vi "DetectIon.vi"(10 "Samples per averaging\nblock":i32=100 min=1 step=1, 11 "Threshold":u32) -> (3 "Ion":bool)   [LabVIEW 2012]
uses:
  <vilib>/DAQmx/read.llb/DAQmx Read (Counter U32 1Chan 1Samp).vi
  <vilib>/DAQmx/create/channels.llb/DAQmx Create Channel (CI-Count Edges).vi
  <vilib>/DAQmx/configure/timing.llb/DAQmx Timing (Sample Clock).vi
  <vilib>/Analysis/baseanly.llb/Mean (DBL).vi
  <vilib>/DAQmx/miscellaneous.llb/DAQmx Fill In Error Info.vi
  <resource>/objmgr/daqmx.rc
  <vilib>/Analysis/NI_AALBase.lvlib
panel:
  out "Mean":dbl format="%0.2f"
  out "Variance":dbl format="%0.2f"
  out "Mean/Variance":dbl
  out "Counts":u32
  in  "Sample rate":dbl=50.0 format="%0.2f"
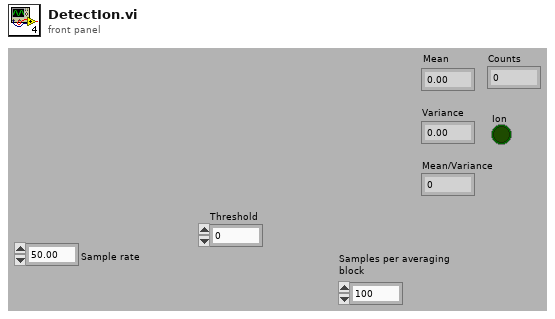
[diagram p1: front panel]
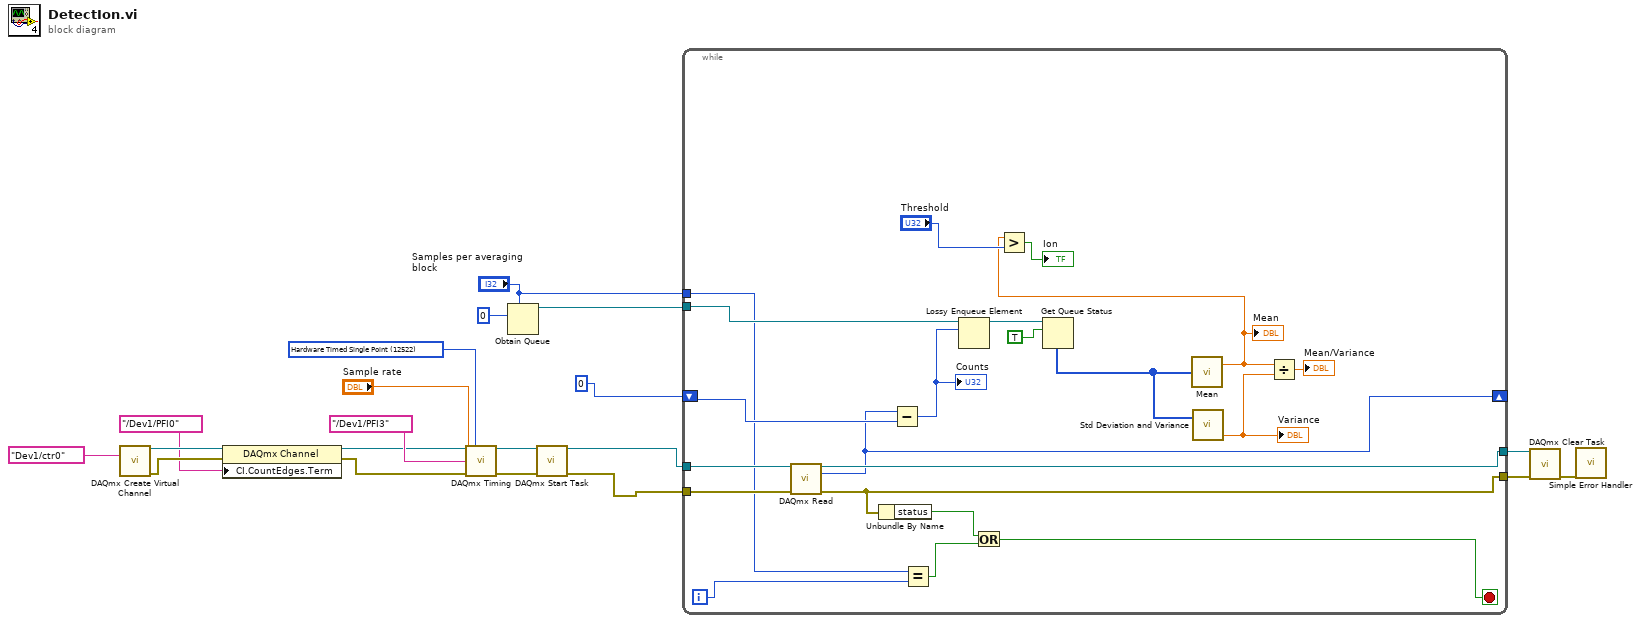
[diagram p0: block diagram]
diagram:
  w9 = 12522 items=["Finite Samples"=10178, "Continuous Samples"=10123, "Hardware Timed Single Point"=12522] ("sample mode")
  n1 = call-poly <vilib>:"DAQmx Create Virtual Channel.vi"("counter"=tag "Dev1/ctr0") -> ("task out"=w14:refnum<k21>, "error out"=w13:errorcluster)  [unwired: 13 in]
  n2 = property class="DAQmx Channel"(reference=w14, error in=w13, "CI.CountEdges.Term"=tag "/Dev1/PFI0") -> (reference out=w16:refnum<k21>, error out=w15:errorcluster)
  n3 = call-poly <vilib>:"DAQmx Timing.vi"("task/channels in"=w16, "sample mode"=w9, "rate"="Sample rate", "source"=tag "/Dev1/PFI3", "error in"=w15) -> ("task out"=w19:refnum<k21>, "error out"=w18:errorcluster)  [unwired: 9 in]
  n4 = Obtain Queue(max queue size (-1, unlimited)="Samples per averaging\nblock", element data type=u32 0) -> (queue out=w4:refnum<queue>)  [unwired: 3 in, 2 out]
  n5 = call <vilib>:"DAQmx Start Task.vi"("task/channels in"=w19, "error in"=w18) -> ("task out"=w2:refnum<k21>, "error out"=w3:errorcluster)  [unwired: 12 in]
  n6 = while {
    tunnel: w4 -> [w32]
    shift-right: [w26] -> _
    shift-left: u32 0 -> [w31]
    tunnel: w2 -> [w30]
    tunnel: w3 -> [w29]
    tunnel: [w28] -> w7
    tunnel: [w27] -> w6
    tunnel: "Samples per averaging\nblock" -> [w23]
    i -> [w24]
    stop <- w21 stop-if-true
    n7 = call-poly <vilib>:"DAQmx Read.vi"("task/channels in"=w30, "error in"=w29) -> ("task out"=w28:refnum<k21>, "data"=w26:u32, "error out"=w27:errorcluster)  [unwired: 11 in]
    n8 = Unbundle By Name(w27) -> ("status"=w41:bool)
    n9 = Subtract(x=w26, y=w31) -> (x-y=w34:u32)
    "Counts" <- w34
    n10 = Equal?(x=w23, y=w24) -> (x = y?=w22:bool)
    n11 = Lossy Enqueue Element(queue=w32, element=w34) -> (queue out=w40:refnum<queue>)  [unwired: 1 in, 3 out]
    n12 = Or(x=w41, y=w22) -> (x .or. y?=w21:bool)
    n13 = Get Queue Status(queue=w40, return elements? (F)=TRUE) -> (elements=w35:u32[])  [unwired: 1 in, 7 out]
    n14 = call-poly <vilib>:"Mean.vi"("X"=w35) -> ("mean"=w33:dbl)  [unwired: 1 out]
    "Mean" <- w33
    n15 = Greater?(x=w33, y="Threshold") -> (0:→"Ion":bool)
    n16 = call <vilib>:"Std Deviation and Variance.vi"("X"=w35) -> ("variance"=w38:dbl)  [unwired: 1 in, 2 out]
    "Variance" <- w38
    n17 = Divide(x=w33, y=w38) -> (x/y=→"Mean/Variance":dbl)
  }
  n18 = call <vilib>:"DAQmx Clear Task.vi"("task in"=w7, "error in"=w6) -> ("error out"=w8:errorcluster)  [unwired: 13 in]
  n19 = call <vilib>:"Simple Error Handler.vi"("error in (no error)"=w8) -> ()  [unwired: 4 in, 5 out]
